vi "Write RespTimeout.vi"(8 "error in (no error)":errorcluster, 10 "RespTimeout":i32, 11 "Picomotor8742Comm in":refnum<class "TCPCommClass.lvclass">) -> (0 "error out":errorcluster, 3 "Picomotor8742Comm out":refnum<class "TCPCommClass.lvclass">)   [LabVIEW 2020, in "TCPCommClass.lvclass"]
uses:
  TCPCommClass.lvclass
  TCPCommClass.lvclass/TCPCommClass.ctl
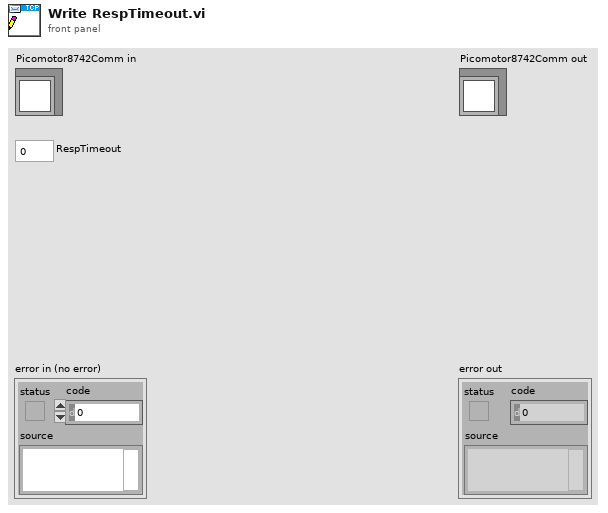
[diagram p1: front panel]
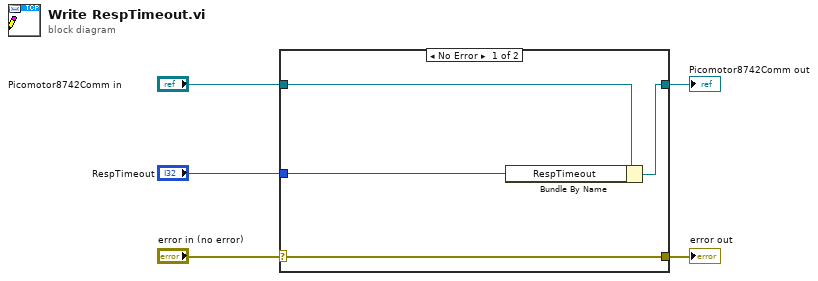
[diagram p0: block diagram]
diagram:
  n1 = case shown="No Error" "error in (no error)" {
    selector: "error in (no error)" -> [w9 w10]
    tunnel: [w9 w10] -> w4
    tunnel: [w7 w11] -> w2
    tunnel: "Picomotor8742Comm in" -> [w8 w11]
    tunnel: "RespTimeout" -> [w6 _]
    frame No Error {
      n2 = Bundle By Name(cluster=w8, "RespTimeout"=w6) -> (w7:refnum<class "TCPCommClass.lvclass">)
    }
    frame Error {
    }
  }
  "error out" <- w4
  "Picomotor8742Comm out" <- w2
